vi "Run Align Data Acquisition.vi"(8 "error in":errorcluster, 9 "Thresholding Cluster 2":T1={"F_DEx"=0, "F_AA"=0, " No of Bins"=100}, 10 "Time Limit":dbl=1.0, 11 "output cluster 2":T2) -> (0 "error out":errorcluster)   [LabVIEW 2009]
uses:
  Acquisition Settings.vi
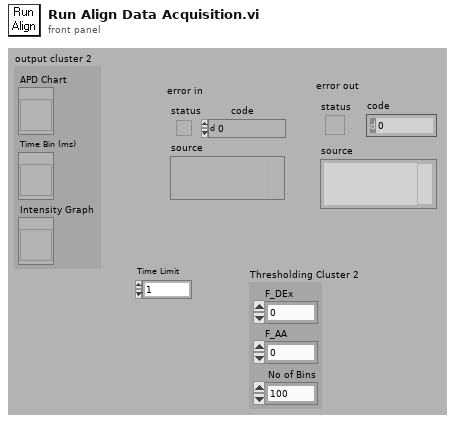
[diagram p1: front panel]
types:
  T1 = cluster{"F_DEx":i32, "F_AA":i32, " No of Bins":i32}
  T2 = cluster{"APD Chart":refnum<vi>, "Time Bin (ms)":refnum<vi>, "Intensity Graph":refnum<vi>}
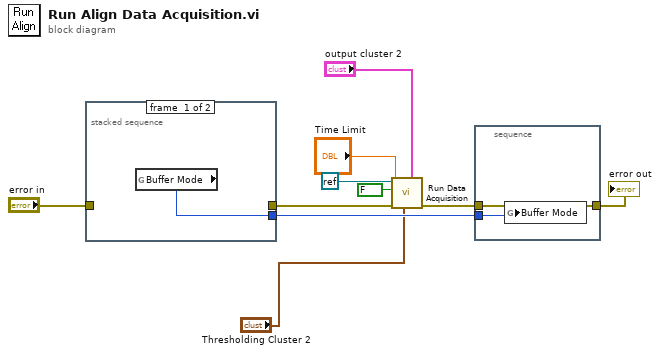
[diagram p0: block diagram]
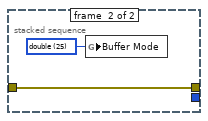
[diagram p2: hidden frame]
diagram:
  n1 = stacked-sequence {
    tunnel: "error in" -> [_ w12]
    tunnel: [_ w12] -> w8
    tunnel: [w11 _] -> w10
    frame #0 {
      n2 = global read "Acquisition Settings.vi" "Buffer Mode"() -> (w11:u32)
    }
    frame #1 {
      w13 = u32 25 items=["yes", "no", "positive", "negative", "high", "low", "low to high", "high to low", "default", "max timebase", "other counter gate", "other counter TC", "other counter output", "other counter source", "source", "gate", "aux line", "in start trigger", "in stop trigger", "automatic", "enabled", "count up", "count down", "hardware", "single", "double", "pulse", "toggle", "quadrature encoder X1", "quadrature encoder X2", "quadrature encoder X4", "two pulse counting", "A high B high", "A high B low", "A low B high", "A low B low", "PFI n", "RTSI n", "timebase n"] ("Buffer Mode")
      n3 = global write "Acquisition Settings.vi" "Buffer Mode"(w13) -> ()
    }
  }
  n4 = call "Run Data Acquisition.vi"("output cluster 2"="output cluster 2", "Thresholding Cluster 2"="Thresholding Cluster 2", "error in (no error)"=w8, "Time Limit"="Time Limit", "Save Data"=FALSE, "refnum in"=refnum<k0> refnum) -> ("error out"=w9:errorcluster)  [unwired: 4 in, 1 out]
  n5 = stacked-sequence {
    tunnel: w9 -> [w14]
    tunnel: w10 -> [w15]
    tunnel: [w14] -> w4
    frame #0 {
      n6 = global write "Acquisition Settings.vi" "Buffer Mode"(w15) -> ()
    }
  }
  "error out" <- w4
